vi "UI cam 1 frame saved.vi"(8 "error in (no error)":errorcluster, 10 "file path":path, 11 "Main_Control in":refnum<class "Main_Control.lvclass">) -> (0 "error out":errorcluster, 3 "Main_Control out":refnum<class "Main_Control.lvclass">)   [LabVIEW 2021, in "Main_Control.lvlib" / "Main_Control.lvclass"]
uses:
  Main_Control.lvclass
  Main_Control.lvclass/Main_Control.ctl
  NI/NI Messages/NI save one frame AI data Msg/NI save one frame AI data Msg.lvclass/NI save one frame AI data Msg.ctl
  <vilib>/ActorFramework/Message Enqueuer/Message Enqueuer.lvclass/Message Enqueuer.ctl
  <vilib>/ActorFramework/Message Enqueuer/Enqueue.vi
  NI/NI Messages/NI save one frame AI data Msg/NI save one frame AI data Msg.lvclass
  C:/Program Files (x86)/National Instruments/LabVIEW 2021/vi.lib/ActorFramework/Message/Message.lvclass
  <vilib>/ActorFramework/Message Priority Queue/Priority Enqueue.vi
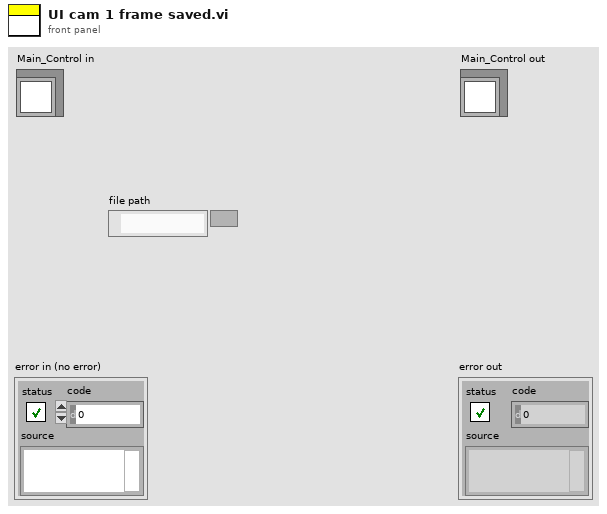
[diagram p1: front panel]
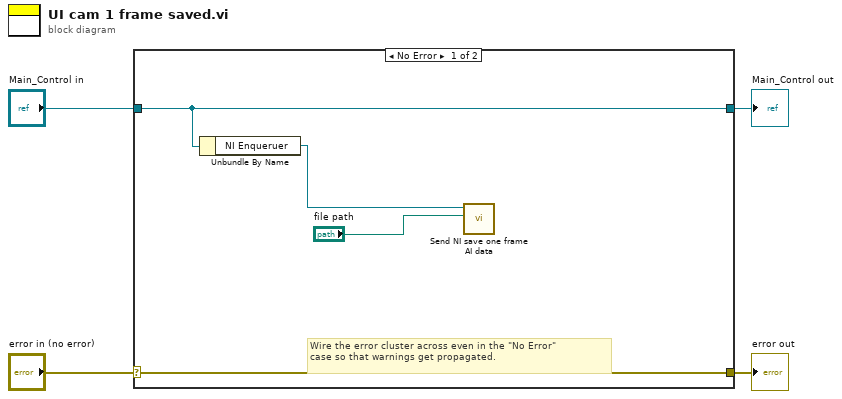
[diagram p0: block diagram]
diagram:
  n1 = case shown="No Error" "error in (no error)" {
    selector: "error in (no error)" -> [w8 w10]
    tunnel: [w8 w10] -> w3
    tunnel: [w6 w9] -> w1
    tunnel: "Main_Control in" -> [w6 w9]
    frame No Error {
      # "Wire the error cluster across even in the \"No Error\"\ncase so that warnings get propagated."
      n2 = Unbundle By Name(w6) -> ("NI Enqueruer"=w5:refnum<class "Message Enqueuer.lvclass">)
      n3 = call "Send NI save one frame AI data.vi"("file path"="file path", "Message Enqueuer"=w5) -> ()  [unwired: 8 in, 2 out]
    }
    frame Error {
    }
  }
  "error out" <- w3
  "Main_Control out" <- w1
